vi "Init Tree.vi"(10 "Settings In":T4={"Step Values"=[], "Only Execute When Test Running"=TRUE, "Reset Sequence When Test Starts"=TRUE, "Current Sequence ID"=0, "Total Iterations"=0, "Current Step Start Timestamp"=0.0, "Number of Sequence Steps"=0, "Num of Analog Channels"=0, "Num of Digital Channels"=0, "Delay Before Starting Sequence"=0.0, "Show UI"=FALSE, "Time Remaining"=0.0, "Test Running"=FALSE, "Pause Timestamp"=0.0, "Default Analog Values"=[], "Default Digital Values"=[]}, 11 "Init Refs":T3) -> (2 "Tree Data":cluster{string[], T1[]} {"?"."Data Type" items=["Tree Parent"=-1, "Numeric"=0, "String"=1, "Boolean"=2, "Enum"=3]}, 3 "Selected Tag":string)   [LabVIEW 2020, in "Sequencer with Output Values.lvlib" / "Sequencer with Output Values.lvclass"]
uses:
  Sequencer with Output Values.lvclass
  Params.ctl
  Step Settings.ctl
  Control Refs.ctl
  Tree Item Settings.ctl
  Data Type.ctl
  Global Tree Data.vi
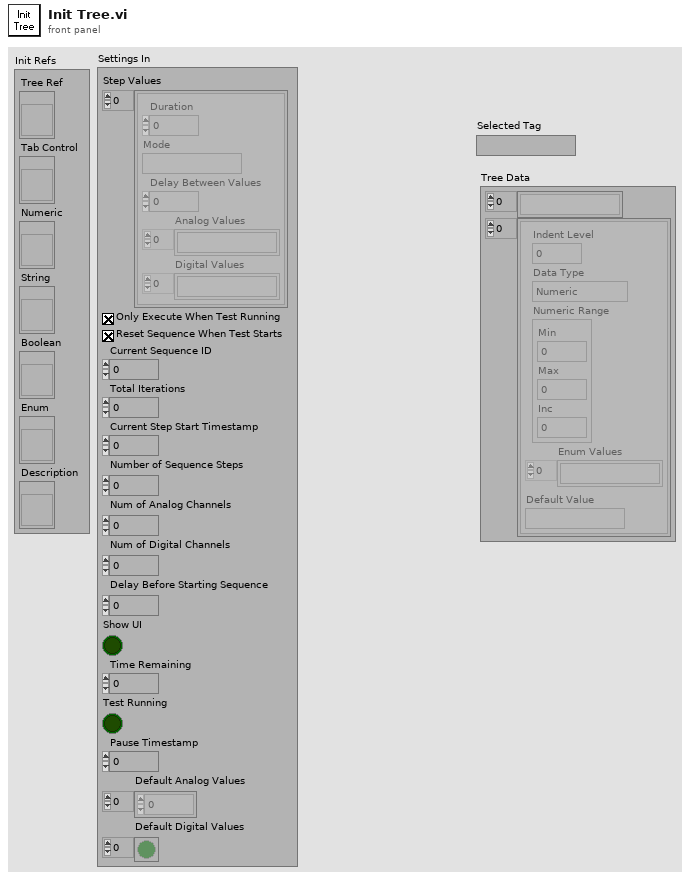
[diagram p1: front panel]
types:
  T1 = typedef "Sequencer with Output Values.lvlib/Sequencer with Output Values.lvclass/Tree Item Settings.ctl" = cluster{"Indent Level":i32, "Data Type":T2, "Numeric Range":cluster{"Min":dbl, "Max":dbl, "Inc":dbl}, "Enum Values":string[], "Default Value":string}
  T2 = typedef "Sequencer with Output Values.lvlib/Sequencer with Output Values.lvclass/Data Type.ctl" = i16
  T3 = typedef "Sequencer with Output Values.lvlib/Sequencer with Output Values.lvclass/Control Refs.ctl" = cluster{"Tree Ref":refnum<vi>, "Tab Control":refnum<vi>, "Numeric":refnum<vi>, "String":refnum<vi>, "Boolean":refnum<vi>, "Enum":refnum<vi>, "Description":refnum<vi>}
  T4 = typedef "Sequencer with Output Values.lvlib/Sequencer with Output Values.lvclass/Params.ctl" = cluster{"Step Values":T5[], "Only Execute When Test Running":bool, "Reset Sequence When Test Starts":bool, "Current Sequence ID":u32, "Total Iterations":u32, "Current Step Start Timestamp":dbl, "Number of Sequence Steps":i32, "Num of Analog Channels":i32, "Num of Digital Channels":i32, "Delay Before Starting Sequence":dbl, "Show UI":bool, "Time Remaining":dbl, "Test Running":bool, "Pause Timestamp":dbl, "Default Analog Values":dbl[], "Default Digital Values":bool[]}
  T5 = typedef "Sequencer with Output Values.lvlib/Sequencer with Output Values.lvclass/Step Settings.ctl" = cluster{"Duration":dbl, "Mode":string, "Delay Between Values":dbl, "Analog Values":string[], "Digital Values":string[]}
  T6 = cluster{"Left Cell String":string, "Child Text":string[], "Child Tag":string, "Item Indent":i32, "Child Only?":bool, "Glyph Index":i32}
  T7 = cluster{"Left Cell String":string, "Child Text":string[], "Child Tag":string, "Item Indent":i32, "Child Only?":bool, "Glyph Index":i32}[]
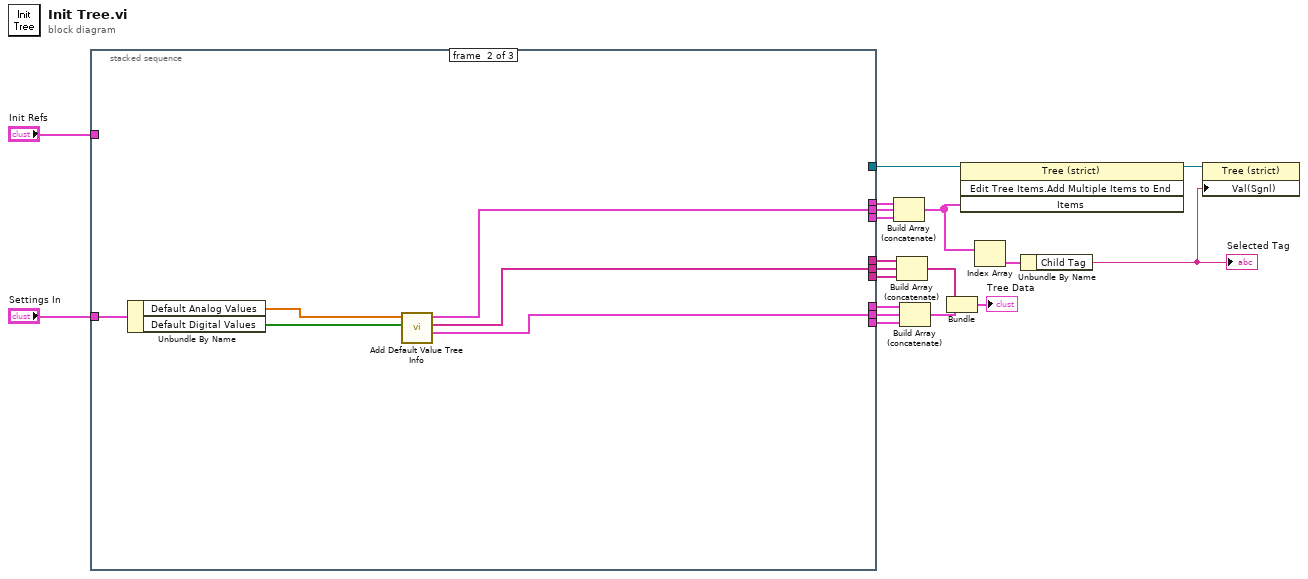
[diagram p0: block diagram]
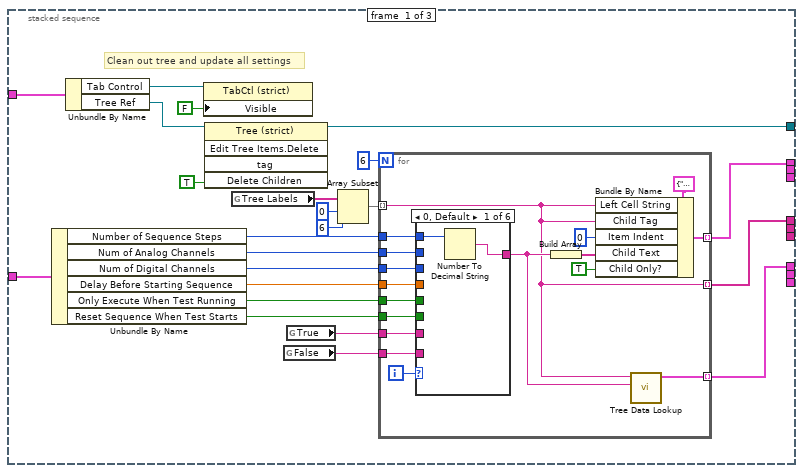
[diagram p2: hidden frame]
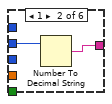
[diagram p3: hidden frame]
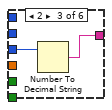
[diagram p4: hidden frame]
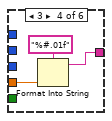
[diagram p5: hidden frame]
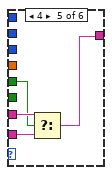
[diagram p6: hidden frame]
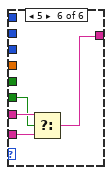
[diagram p7: hidden frame]
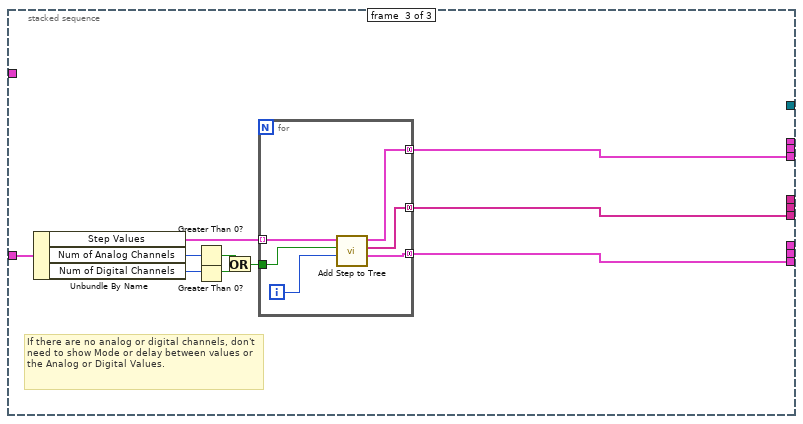
[diagram p8: hidden frame]
diagram:
  n1 = stacked-sequence {
    tunnel: "Init Refs" -> [w40 _ _]
    tunnel: "Settings In" -> [w37 w82 w92]
    tunnel: [_ _ w88] -> w6
    tunnel: [w27 _ _] -> w17
    tunnel: [w26 _ _] -> w16
    tunnel: [w25 _ _] -> w11
    tunnel: [w24 _ _] -> w9
    tunnel: [_ _ w87] -> w5
    tunnel: [_ _ w86] -> w4
    tunnel: [_ w79 _] -> w3
    tunnel: [_ w78 _] -> w2
    tunnel: [_ w77 _] -> w1
    frame #0 {
      # "Clean out tree and update all settings"
      n2 = Unbundle By Name(w37) -> ("Number of Sequence Steps"=w35:i32, "Num of Analog Channels"=w34:i32, "Num of Digital Channels"=w33:i32, "Delay Before Starting Sequence"=w32:dbl, "Only Execute When Test Running"=w31:bool, "Reset Sequence When Test Starts"=w30:bool)
      n3 = Unbundle By Name(w40) -> ("Tab Control"=w39:refnum<vi>, "Tree Ref"=w42:refnum<vi>)
      n4 = property class="TabCtl (strict)"(reference=w39, "Visible"=FALSE) -> ()  [unwired: 1 in, 2 out]
      n5 = invoke class="Tree (strict)" method="Edit Tree Items.Delete"(reference=w42, "Delete Children"=TRUE ("Delete Children?")) -> (reference out=w26:refnum<vi>)  [unwired: 3 in, 4 out]
      n6 = global read "Global Tree Data.vi" "Tree Labels"() -> (w23:string[])
      n7 = global read "Global Tree Data.vi" "False"() -> (w28:string)
      n8 = global read "Global Tree Data.vi" "True"() -> (w29:string)
      n9 = Array Subset(array=w23, index=0, length=6) -> (w20:string[])
      n10 = for {
        N: 6 -> [_]
        tunnel: w20 -> [w43] mode=indexing
        tunnel: w35 -> [w57]
        tunnel: w34 -> [w56]
        tunnel: w33 -> [w55]
        tunnel: w32 -> [w54]
        tunnel: w31 -> [w53]
        tunnel: w30 -> [w52]
        tunnel: w29 -> [w49]
        tunnel: w28 -> [w48]
        tunnel: [w47] -> w27 mode=indexing
        tunnel: [w44] -> w25 mode=indexing
        tunnel: [w43] -> w24 mode=indexing
        i -> [w50]
        n11 = case shown="0, Default" w50 {
          tunnel: w57 -> [w61 _ _ _ _ _]
          tunnel: w56 -> [_ w63 _ _ _ _]
          tunnel: w55 -> [_ _ w65 _ _ _]
          tunnel: w54 -> [_ _ _ w67 _ _]
          tunnel: w53 -> [_ _ _ _ w70 _]
          tunnel: w52 -> [_ _ _ _ _ w73]
          tunnel: [w60 w62 w64 w66 w69 w74] -> w45
          tunnel: w49 -> [_ _ _ _ w72 w76]
          tunnel: w48 -> [_ _ _ _ w71 w75]
          frame 0, Default {
            n12 = Number To Decimal String(number=w61) -> (decimal integer string=w60:string)  [unwired: 1 in]
          }
          frame 1 {
            n13 = Number To Decimal String(number=w63) -> (decimal integer string=w62:string)  [unwired: 1 in]
          }
          frame 2 {
            n14 = Number To Decimal String(number=w65) -> (decimal integer string=w64:string)  [unwired: 1 in]
          }
          frame 3 {
            n15 = Format Into String(format string="%#.01f", w67) -> (resulting string=w66:string)  [unwired: 2 in, 1 out]
          }
          frame 4 {
            n16 = Select(t=w72, s=w70, f=w71) -> (s? t:f=w69:string)
          }
          frame 5 {
            n17 = Select(t=w76, s=w73, f=w75) -> (s? t:f=w74:string)
          }
        }
        n18 = Build Array(w45) -> (w51:string[])
        n19 = Bundle By Name(cluster=T6 {"Left Cell String"="", "Child Text"=[], "Child Tag"="", "Item Indent"=0, "Child Only?"=FALSE, "Glyph Index"=0} ("Item"), "Left Cell String"=w43, "Child Tag"=w43, "Item Indent"=0, "Child Text"=w51, "Child Only?"=TRUE) -> (w47:T6)
        n20 = call "Tree Data Lookup.vi"("Value"=w45, "Key"=w43) -> ("Tree Data"=w44:T1)  [unwired: 9 in]
      }
    }
    frame #1 {
      n21 = Unbundle By Name(w82) -> ("Default Analog Values"=w81:dbl[], "Default Digital Values"=w80:bool[])
      n22 = call "Add Default Value Tree Info.vi"("Default Digital Values"=w80, "Default Analog Values"=w81) -> ("Tree Data"=w77:T1[], "Tags"=w78:string[], "Tree Items"=w79:T7)  [unwired: 7 in]
    }
    frame #2 {
      # "If there are no analog or digital channels, don't need to show Mode or delay between values or the Analog or Digital Values."
      n23 = Unbundle By Name(w92) -> ("Step Values"=w90:T5[], "Num of Analog Channels"=w91:i32, "Num of Digital Channels"=w89:i32)
      n24 = Greater Than 0?(x=w91) -> (x > 0?=w85:bool)
      n25 = Greater Than 0?(x=w89) -> (x > 0?=w84:bool)
      n26 = Or(x=w85, y=w84) -> (x .or. y?=w83:bool)
      n27 = for {
        tunnel: w90 -> [w98] mode=indexing
        tunnel: [w95] -> w88 mode=concatenating
        tunnel: [w94] -> w87 mode=concatenating
        tunnel: [w93] -> w86 mode=concatenating
        tunnel: w83 -> [w97]
        i -> [w96]
        n28 = call "Add Step to Tree.vi"("Step Index"=w96, "Channels Defined"=w97, "Step Settings"=w98) -> ("Tree Data"=w93:T1[], "Tree Tags"=w94:string[], "Tree Items"=w95:T7)  [unwired: 6 in]
      }
    }
  }
  n29 = Build Array (concatenate)(w17, w3, w6) -> (w15:T7)
  n30 = Build Array (concatenate)(w9, w2, w5) -> (w8:string[])
  n31 = Build Array (concatenate)(w11, w1, w4) -> (w10:T1[])
  n32 = Bundle(w8, w10) -> (→"Tree Data":cluster{string[], T1[]})  [unwired: 1 in]
  n33 = invoke class="Tree (strict)" method="Edit Tree Items.Add Multiple Items to End"(reference=w16, "Items"=w15) -> (reference out=w13:refnum<vi>)  [unwired: 2 in, 3 out]
  n34 = Index Array(array=w15) -> (element=w14:T6)  [unwired: 1 in]
  n35 = Unbundle By Name(w14) -> ("Child Tag"=w12:string)
  "Selected Tag" <- w12
  n36 = property class="Tree (strict)"(reference=w13, "Val(Sgnl)"=w12) -> ()  [unwired: 1 in, 2 out]
